vi "Read VI Blocks.vi"(8 "error in (no error)":errorcluster, 11 "Path in (vi, ctl, llb)":path) -> (0 "error out":errorcluster, 1 "Filenames":string[](array[string]), 2 "Blocks":T1(array[cluster]), 3 "Path out":path)   [LabVIEW 2022 SP3]
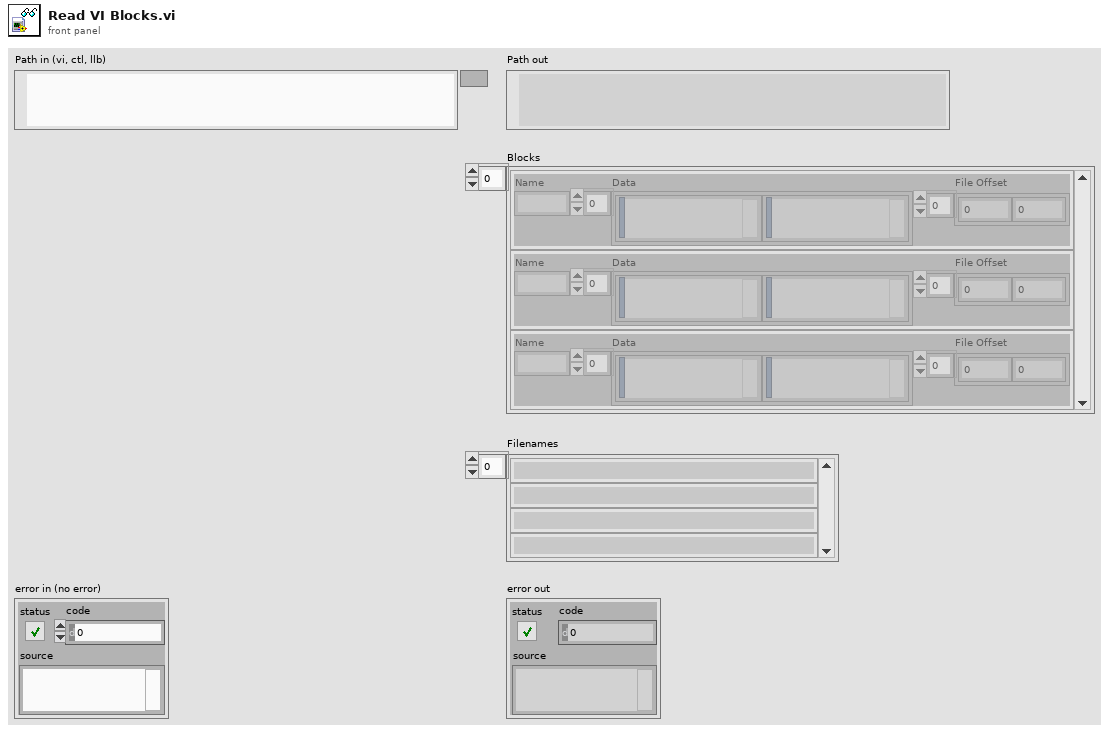
[diagram p1: front panel]
types:
  T1 = cluster{"Name":string, "Data":string[], "File Offset":u32[]}[]
  T2 = cluster{"BLOCK_INFO":cluster{"Int1":i32, "Int2":i32, "Int3":i32, "Offset":u32, "Size":u32}[]}
  T3 = cluster{"Name":string, "Data":string[], "Offset":u32[]}
  T4 = enum16{"open", "replace", "create", "open or create", "replace or create", "replace or create with confirmation"}
  T5 = cluster{"RSRC_Identifier":u64, "RSRC_Type":u32, "RSRC_Creator":u32, "Info_Offset":u32, "Info_Size":u32, "Data_Offset":u32, "Data_Size":u32}
  T6 = cluster{"Int1":i32, "Int2":i32, "Int3":i32, "Offset":u32, "Size":u32}
  T7 = cluster{"Int1":i32, "Int2":i32, "Int3":i32, "Offset":u32, "Size":u32}[]
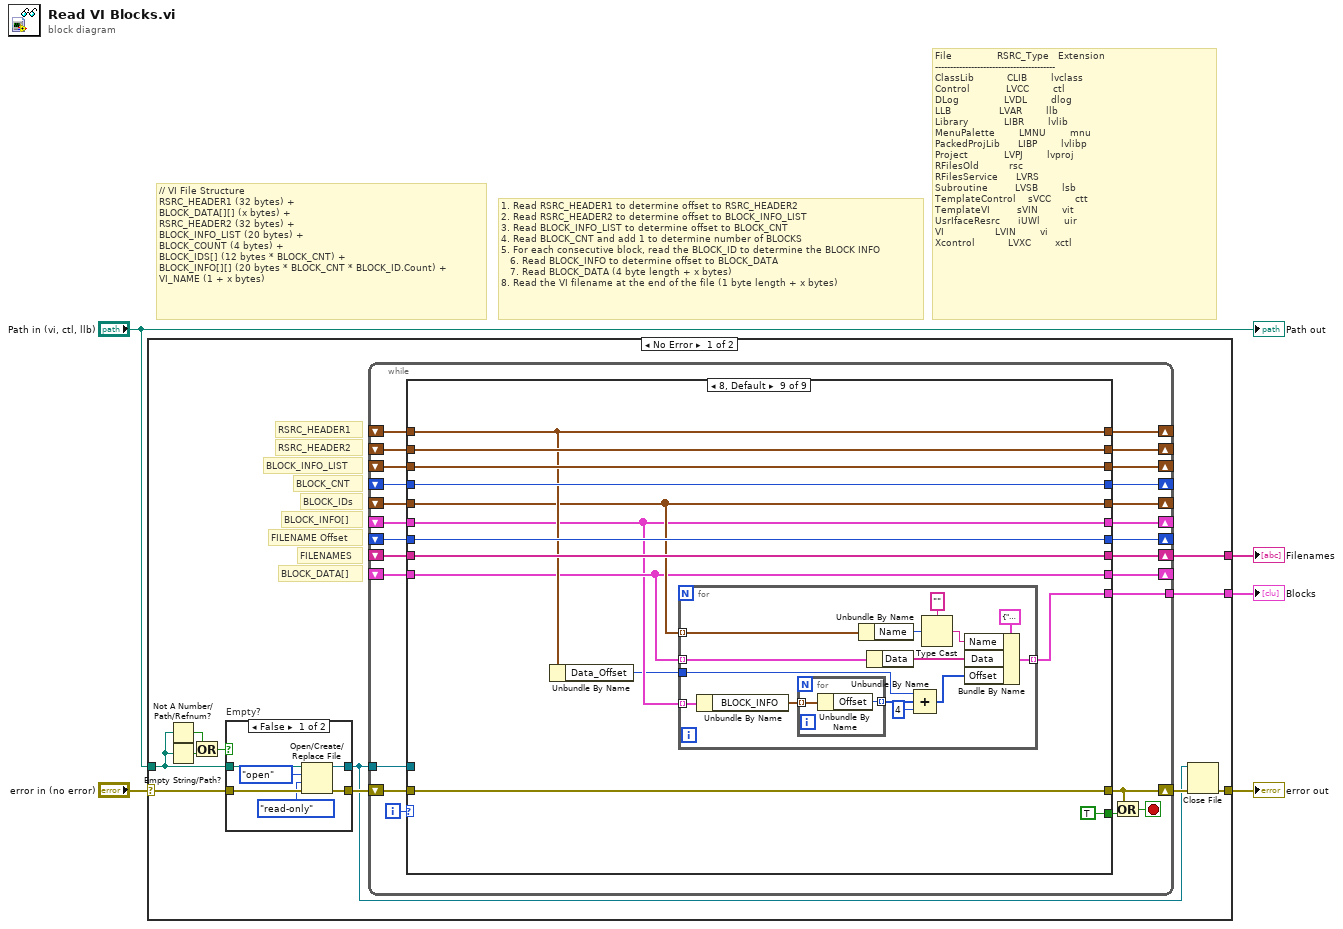
[diagram p0: block diagram]
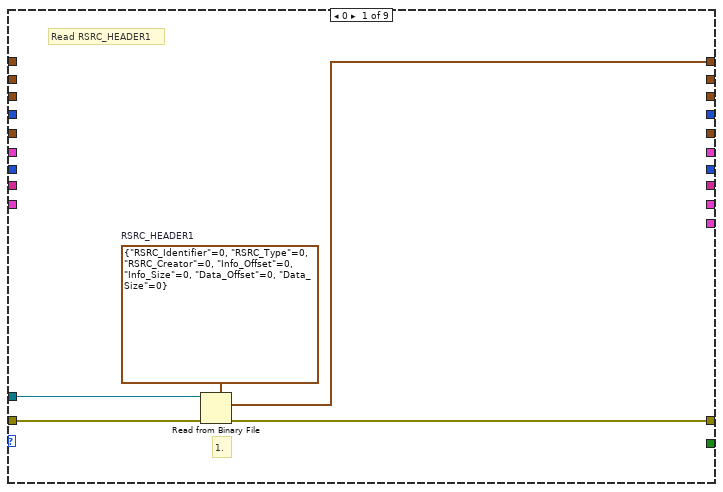
[diagram p2: hidden frame]
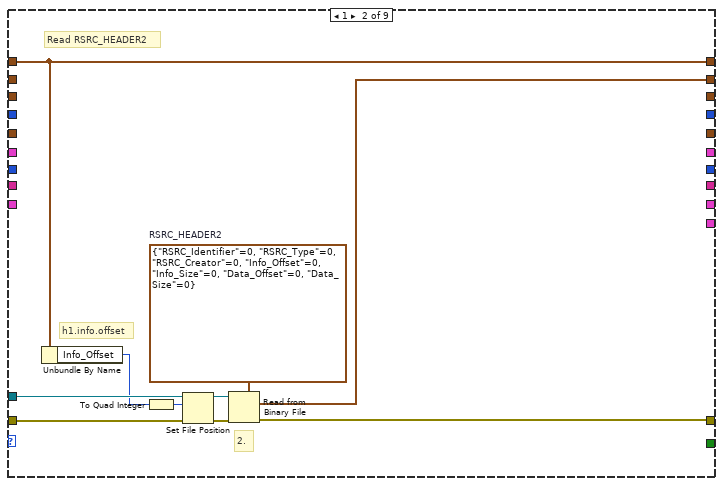
[diagram p3: hidden frame]
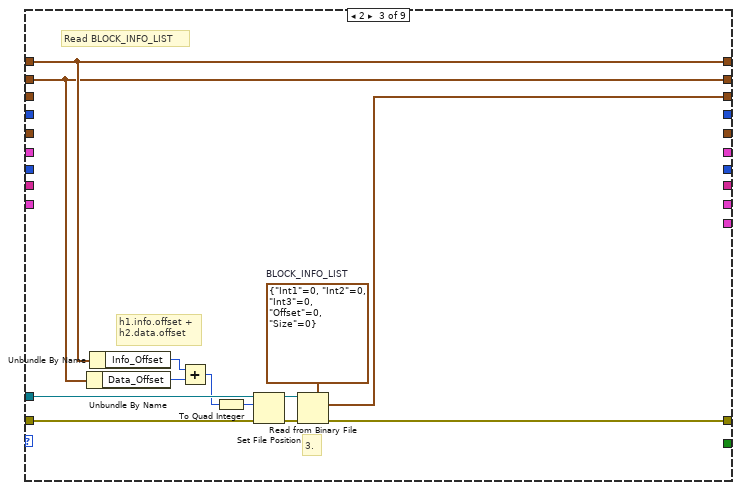
[diagram p4: hidden frame]
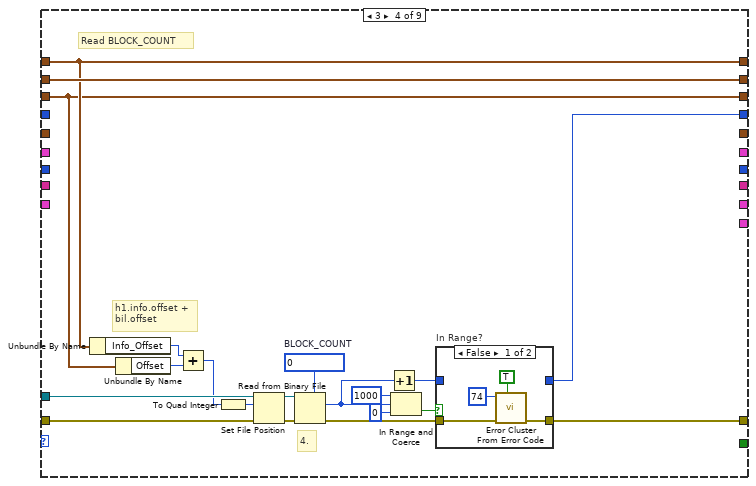
[diagram p5: hidden frame]
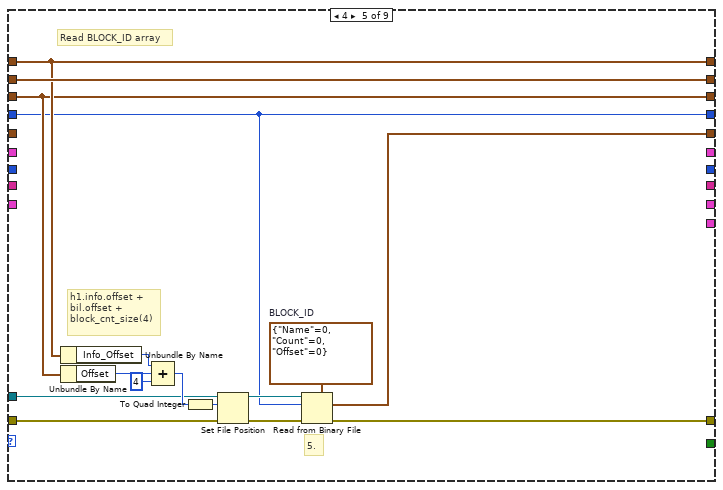
[diagram p7: hidden frame]
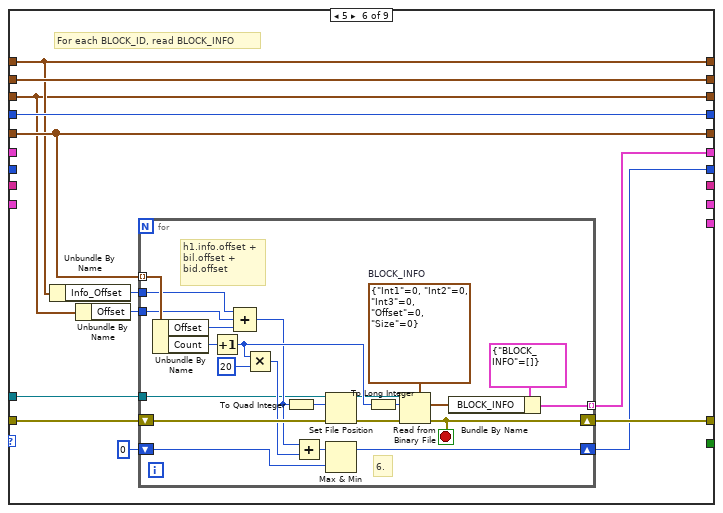
[diagram p8: hidden frame]
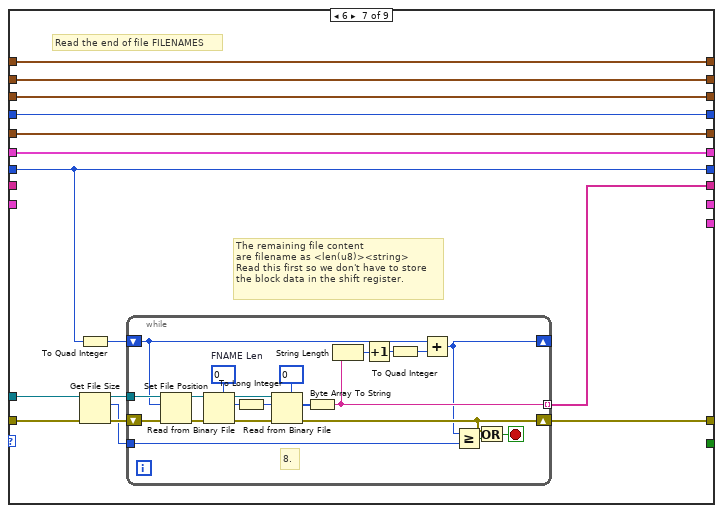
[diagram p9: hidden frame]
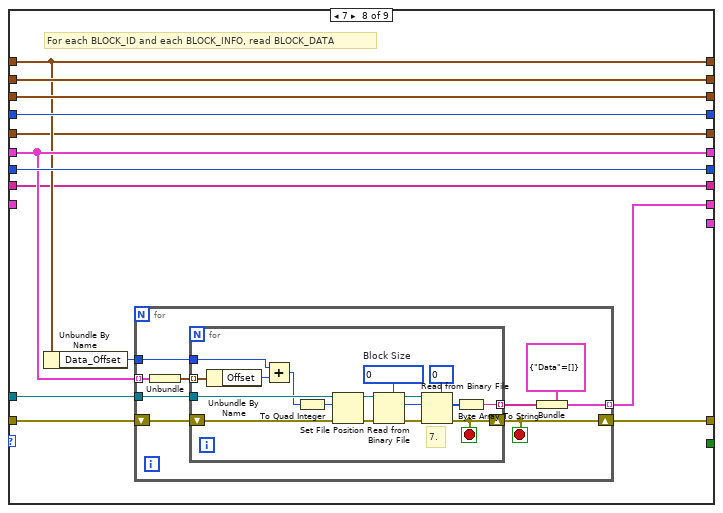
[diagram p10: hidden frame]
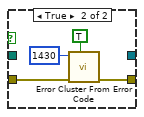
[diagram p11: hidden frame]
diagram:
  # "1. Read RSRC_HEADER1 to determine offset to RSRC_HEADER2\n2. Read RSRC_HEADER2 to determine offset to BLOCK_INFO_LIST\n3. Read BLOCK_INFO_LIST to determine offset to BLOCK_CNT\n4. Read BLOCK_CNT and add 1 to determine number of BLOCKS\n5. For each consecutive block, read the BLOCK_ID to determine the BLOCK INFO\n   6. Read BLOCK_INFO to determine offset to BLOCK_DATA\n   7. Read BLOCK_DATA (4 byte length + x bytes)\n8. Read the VI filename at the end of the file (1 byte length + x bytes)"
  # "// VI File Structure\nRSRC_HEADER1 (32 bytes) + \nBLOCK_DATA[][] (x bytes) +\nRSRC_HEADER2 (32 bytes) + \nBLOCK_INFO_LIST (20 bytes) +\nBLOCK_COUNT (4 bytes) + \nBLOCK_IDS[] (12 bytes * BLOCK_CNT) +\nBLOCK_INFO[][] (20 bytes * BLOCK_CNT * BLOCK_ID.Count) +\nVI_NAME (1 + x bytes)"
  # "File               RSRC_Type   Extension\n----------------------------------------\nClassLib           CLIB        lvclass\nControl            LVCC        ctl\nDLog               LVDL        dlog\nLLB                LVAR        llb\nLibrary            LIBR        lvlib\nMenuPalette        LMNU        mnu\nPackedProjLib      LIBP        lvlibp\nProject            LVPJ        lvproj\nRFilesOld          rsc         \nRFilesService      LVRS        \nSubroutine         LVSB        lsb\nTemplateControl    sVCC        ctt\nTemplateVI         sVIN        vit\nUsrIfaceResrc      iUWl        uir\nVI                 LVIN        vi\nXcontrol           LVXC        xctl"
  n1 = case shown="No Error" "error in (no error)" {
    selector: "error in (no error)" -> [w16 w262]
    tunnel: "Path in (vi, ctl, llb)" -> [w15 _]
    tunnel: [w11 _] -> w4
    tunnel: [w8 w262] -> w3
    tunnel: [w6 _] -> w2
    frame No Error {
      # "BLOCK_DATA[]"
      # "FILENAME Offset"
      # "BLOCK_INFO[]"
      # "BLOCK_IDs"
      # "BLOCK_CNT"
      # "BLOCK_INFO_LIST"
      # "RSRC_HEADER2"
      # "FILENAMES"
      # "RSRC_HEADER1"
      n2 = Not A Number/Path/Refnum?(number/path/refnum=w15) -> (NaN/Path/Refnum?=w13:bool)
      n3 = Empty String/Path?(string/path=w15) -> (empty?=w14:bool)
      n4 = Or(x=w13, y=w14) -> (x .or. y?=w12:bool)
      n5 = case "Empty?" shown="False" w12 {
        tunnel: w16 -> [w257 w261]
        tunnel: w15 -> [w254 _]
        tunnel: [w253 w258] -> w10
        tunnel: [w252 _] -> w7
        frame False {
          n6 = Open/Create/Replace File(file path (use dialog)=w254, error in=w257, operation (0:open)=T4."open", access (0:read/write)=enum16{"read/write", "read-only", "write-only"}."read-only") -> (refnum out=w252:refnum<file>, error out=w253:errorcluster)  [unwired: 2 in, 1 out]
        }
        frame True {
          n7 = call <vilib>:"Error Cluster From Error Code.vi"("show call chain? (False)"=TRUE, "error in (no error)"=w261, "error code (0)"=1430) -> ("error out"=w258:errorcluster)  [unwired: 6 in]
        }
      }
      n8 = while {
        tunnel: w7 -> [w40]
        shift-right: [w36] -> w9
        shift-left: w10 -> [w41]
        shift-right: [w38] -> _
        shift-left: _ -> [w37]
        shift-right: [w33] -> _
        shift-left: _ -> [w32]
        shift-right: [w31] -> _
        shift-left: _ -> [w30]
        shift-right: [w29] -> _
        shift-left: _ -> [w28]
        shift-right: [w27] -> _
        shift-left: _ -> [w26]
        shift-right: [w25] -> _
        shift-left: _ -> [w24]
        shift-right: [w23] -> _
        shift-left: _ -> [w22]
        shift-right: [w20] -> w11
        shift-left: _ -> [w19]
        shift-right: [w21] -> _
        shift-left: _ -> [w18]
        tunnel: [w17] -> w6
        i -> [w39]
        stop <- w35 stop-if-true
        n9 = case shown="8, Default" w39 {
          tunnel: w41 -> [w46 w56 w69 w85 w108 w122 w156 w192 w229]
          tunnel: [w44 w54 w68 w84 w107 w120 w155 w186 w229] -> w36
          tunnel: w40 -> [w45 w51 w61 w74 w99 w121 w152 w188 _]
          tunnel: [w42 w55 w67 w83 w106 w118 w162 w190 w228] -> w38
          tunnel: w37 -> [_ w55 w67 w83 w106 w118 w162 w190 w228]
          tunnel: [_ _ _ _ _ _ _ _ TRUE] -> w34
          tunnel: [_ w53 w66 w89 w111 w124 w161 w196 w235] -> w33
          tunnel: w32 -> [_ _ w66 w89 w111 w124 w161 w196 w235]
          tunnel: [_ _ w63 w82 w105 w117 w160 w195 w234] -> w31
          tunnel: w30 -> [_ _ _ w82 w105 w117 w160 w195 w234]
          tunnel: [_ _ _ w76 w97 w123 w159 w194 w233] -> w29
          tunnel: w28 -> [_ _ _ _ w97 w123 w159 w194 w233]
          tunnel: [_ _ _ _ w96 w119 w158 w187 w227] -> w27
          tunnel: w26 -> [_ _ _ _ _ w119 w158 w187 w227]
          tunnel: [_ _ _ _ _ w113 w157 w191 w224] -> w25
          tunnel: w24 -> [_ _ _ _ _ _ w157 w191 w224]
          tunnel: [_ _ _ _ _ w112 w150 w193 w232] -> w23
          tunnel: w22 -> [_ _ _ _ _ _ w150 w193 w232]
          tunnel: [_ _ _ _ _ _ _ w185 w226] -> w21
          tunnel: [_ _ _ _ _ _ w154 w184 w231] -> w20
          tunnel: w19 -> [_ _ _ _ _ _ _ w184 w231]
          tunnel: w18 -> [_ _ _ _ _ _ _ _ w226]
          tunnel: [_ _ _ _ _ _ _ _ w225] -> w17
          frame 0 {
            w43 = T5 {"RSRC_Identifier"=0, "RSRC_Type"=0, "RSRC_Creator"=0, "Info_Offset"=0, "Info_Size"=0, "Data_Offset"=0, "Data_Size"=0}  # RSRC_HEADER1
            # "Read RSRC_HEADER1"
            # "1."
            n10 = Read from Binary File(5:w43, 8:w46, 11:w45) -> (0:w44:errorcluster, 2:w42:T5)  [unwired: 3 in, 2 out]
          }
          frame 1 {
            w49 = T5 {"RSRC_Identifier"=0, "RSRC_Type"=0, "RSRC_Creator"=0, "Info_Offset"=0, "Info_Size"=0, "Data_Offset"=0, "Data_Size"=0}  # RSRC_HEADER2
            # "Read RSRC_HEADER2"
            # "2."
            # "h1.info.offset"
            n11 = Unbundle By Name(w55) -> ("Info_Offset"=w50:u32)
            n12 = To Quad Integer(1:w50) -> (0:w47:i64)
            n13 = Set File Position(offset (in bytes) (0)=w47, refnum=w51, error in=w56) -> (refnum out=w48:refnum<file>, error out=w52:errorcluster)  [unwired: 1 in]
            n14 = Read from Binary File(5:w49, 8:w52, 11:w48) -> (0:w54:errorcluster, 2:w53:T5)  [unwired: 3 in, 2 out]
          }
          frame 2 {
            w60 = T6 {"Int1"=0, "Int2"=0, "Int3"=0, "Offset"=0, "Size"=0}  # BLOCK_INFO_LIST
            # "Read BLOCK_INFO_LIST"
            # "3."
            # "h1.info.offset +\nh2.data.offset"
            n15 = Unbundle By Name(w66) -> ("Data_Offset"=w65:u32)
            n16 = Unbundle By Name(w67) -> ("Info_Offset"=w64:u32)
            n17 = Add(x=w64, y=w65) -> (x+y=w58:u32)
            n18 = To Quad Integer(1:w58) -> (0:w57:i64)
            n19 = Set File Position(offset (in bytes) (0)=w57, refnum=w61, error in=w69) -> (refnum out=w59:refnum<file>, error out=w62:errorcluster)  [unwired: 1 in]
            n20 = Read from Binary File(5:w60, 8:w62, 11:w59) -> (0:w68:errorcluster, 2:w63:T6)  [unwired: 3 in, 2 out]
          }
          frame 3 {
            w73 = 0  # BLOCK_COUNT
            # "Read BLOCK_COUNT"
            # "4."
            # "h1.info.offset +\nbil.offset"
            n21 = Unbundle By Name(w83) -> ("Info_Offset"=w80:u32)
            n22 = Unbundle By Name(w82) -> ("Offset"=w81:u32)
            n23 = Add(x=w80, y=w81) -> (x+y=w71:u32)
            n24 = To Quad Integer(1:w71) -> (0:w70:i64)
            n25 = Set File Position(offset (in bytes) (0)=w70, refnum=w74, error in=w85) -> (refnum out=w72:refnum<file>, error out=w75:errorcluster)  [unwired: 1 in]
            n26 = Read from Binary File(5:w73, 8:w75, 11:w72) -> (0:w86:errorcluster, 2:w77:i32)  [unwired: 3 in, 2 out]
            n27 = Increment(x=w77) -> (x+1=w78:i32)
            n28 = In Range and Coerce(upper limit=1000, x=w77, lower limit=0) -> (In Range?=w79:bool)  [unwired: 1 out]
            n29 = case "In Range?" shown="False" w79 {
              tunnel: w86 -> [w91 w95]
              tunnel: [w90 w95] -> w84
              tunnel: w78 -> [_ w94]
              tunnel: [_ w94] -> w76
              frame False {
                n30 = call <vilib>:"Error Cluster From Error Code.vi"("show call chain? (False)"=TRUE, "error in (no error)"=w91, "error code (0)"=74) -> ("error out"=w90:errorcluster)  [unwired: 6 in]
              }
              frame True {
              }
            }
          }
          frame 4 {
            w101 = cluster{"Name":u32, "Count":u32, "Offset":u32} {"Name"=0, "Count"=0, "Offset"=0}  # BLOCK_ID
            # "Read BLOCK_ID array"
            # "5."
            # "h1.info.offset +\nbil.offset +\nblock_cnt_size(4)"
            n31 = Unbundle By Name(w106) -> ("Info_Offset"=w110:u32)
            n32 = Unbundle By Name(w105) -> ("Offset"=w109:u32)
            n33 = Compound Arithmetic op=ADD(w110, w109, u32 4 ("value")) -> (w100:u32)
            n34 = To Quad Integer(1:w100) -> (0:w98:i64)
            n35 = Set File Position(offset (in bytes) (0)=w98, refnum=w99, error in=w108) -> (refnum out=w102:refnum<file>, error out=w103:errorcluster)  [unwired: 1 in]
            n36 = Read from Binary File(5:w101, 8:w103, 10:w97, 11:w102) -> (0:w107:errorcluster, 2:w96:cluster{"Name":u32, "Count":u32, "Offset":u32}[])  [unwired: 2 in, 2 out]
          }
          frame 5 {
            # "For each BLOCK_ID, read BLOCK_INFO"
            n37 = Unbundle By Name(w118) -> ("Info_Offset"=w116:u32)
            n38 = Unbundle By Name(w117) -> ("Offset"=w115:u32)
            n39 = for {
              tunnel: w121 -> [w127]
              shift-right: [w134] -> w120
              shift-left: w122 -> [w147]
              tunnel: w119 -> [w146] mode=indexing
              tunnel: w116 -> [w142]
              tunnel: w115 -> [w141]
              shift-right: [w138] -> w112
              shift-left: u32 0 -> [w137]
              tunnel: [w135] -> w113 mode=indexing
              stop <- w134 stop-if-true
              w133 = T6 {"Int1"=0, "Int2"=0, "Int3"=0, "Offset"=0, "Size"=0}  # BLOCK_INFO
              # "6."
              # "h1.info.offset +\nbil.offset +\nbid.offset"
              n40 = Unbundle By Name(w146) -> ("Offset"=w143:u32, "Count"=w144:u32)
              n41 = Increment(x=w144) -> (x+1=w132:u32)
              n42 = Compound Arithmetic op=ADD(w142, w141, w143) -> (w128:u32)
              n43 = Multiply(x=w132, y=u32 20 ("length (rest)")) -> (x*y=w140:u32)
              n44 = To Quad Integer(1:w128) -> (0:w126:i64)
              n45 = Add(x=w128, y=w140) -> (x+y=w139:u32)
              n46 = Set File Position(offset (in bytes) (0)=w126, refnum=w127, error in=w147) -> (refnum out=w130:refnum<file>, error out=w131:errorcluster)  [unwired: 1 in]
              n47 = Max & Min(x=w139, y=w137) -> (max(x,y)=w138:u32)  [unwired: 1 out]
              n48 = To Long Integer(number=w132) -> (32bit integer=w129:i32)
              n49 = Read from Binary File(5:w133, 8:w131, 10:w129, 11:w130) -> (0:w134:errorcluster, 2:w136:T7)  [unwired: 2 in, 2 out]
              n50 = Bundle By Name(cluster=T2 {"BLOCK_INFO"=[]}, "BLOCK_INFO"=w136) -> (w135:T2)
            }
          }
          frame 6 {
            # "Read the end of file FILENAMES"
            # "The remaining file content\nare filename as <len(u8)><string>\nRead this first so we don't have to store\nthe block data in the shift register."
            n51 = To Quad Integer(1:w150) -> (0:w149:i64)
            n52 = Get File Size(file=w152, error in=w156) -> (refnum out=w151:refnum<file>, size (in bytes)=w148:i64, 0:w153:errorcluster)
            n53 = while {
              tunnel: [w172] -> w154 mode=indexing
              tunnel: w151 -> [w181]
              shift-right: [w170] -> w155
              shift-left: w153 -> [w183]
              shift-right: [w165] -> _
              shift-left: w149 -> [w166]
              tunnel: w148 -> [w164]
              stop <- w169 stop-if-true
              w178 = u8 0  # FNAME Len
              # "8."
              n54 = Set File Position(offset (in bytes) (0)=w166, refnum=w181, error in=w183) -> (refnum out=w180:refnum<file>, error out=w182:errorcluster)  [unwired: 1 in]
              n55 = Read from Binary File(5:w178, 8:w182, 11:w180) -> (0:w179:errorcluster, 2:w175:u8, 3:w176:refnum<file>)  [unwired: 3 in, 1 out]
              n56 = To Long Integer(number=w175) -> (32bit integer=w174:i32)
              n57 = Read from Binary File(5:u8 0, 8:w179, 10:w174, 11:w176) -> (0:w170:errorcluster, 2:w173:u8[])  [unwired: 2 in, 2 out]
              n58 = Byte Array To String(unsigned byte array=w173) -> (string=w172:string)
              n59 = String Length(string=w172) -> (length=w171:i32)
              n60 = Increment(x=w171) -> (x+1=w168:i32)
              n61 = To Quad Integer(1:w168) -> (0:w167:i64)
              n62 = Add(x=w166, y=w167) -> (x+y=w165:i64)
              n63 = Greater Or Equal?(x=w165, y=w164) -> (x >= y?=w163:bool)
              n64 = Or(x=w170, y=w163) -> (x .or. y?=w169:bool)
            }
          }
          frame 7 {
            # "For each BLOCK_ID and each BLOCK_INFO, read BLOCK_DATA"
            n65 = Unbundle By Name(w190) -> ("Data_Offset"=w189:u32)
            n66 = for {
              tunnel: w191 -> [w204] mode=indexing
              tunnel: w189 -> [w202]
              tunnel: w188 -> [w201]
              shift-right: [w200] -> w186
              shift-left: w192 -> [w205]
              tunnel: [w198] -> w185 mode=indexing
              stop <- w200 stop-if-true
              n67 = Unbundle(w204) -> ("BLOCK_INFO"=w203:T7)
              n68 = for {
                tunnel: w201 -> [w215]
                shift-right: [w217] -> w200
                shift-left: w205 -> [w222]
                tunnel: [w206] -> w199 mode=indexing
                tunnel: w203 -> [w219] mode=indexing
                tunnel: w202 -> [w218]
                stop <- w217 stop-if-true
                w209 = 0  # Block Size
                # "7."
                n69 = Unbundle By Name(w219) -> ("Offset"=w221:u32)
                n70 = Add(x=w218, y=w221) -> (x+y=w214:u32)
                n71 = To Quad Integer(1:w214) -> (0:w213:i64)
                n72 = Set File Position(offset (in bytes) (0)=w213, refnum=w215, error in=w222) -> (refnum out=w211:refnum<file>, error out=w216:errorcluster)  [unwired: 1 in]
                n73 = Read from Binary File(5:w209, 8:w216, 11:w211) -> (0:w212:errorcluster, 2:w207:i32, 3:w210:refnum<file>)  [unwired: 3 in, 1 out]
                n74 = Read from Binary File(5:u8 0, 8:w212, 10:w207, 11:w210) -> (0:w217:errorcluster, 2:w220:u8[])  [unwired: 2 in, 2 out]
                n75 = Byte Array To String(unsigned byte array=w220) -> (string=w206:string)
              }
              n76 = Bundle(cluster=cluster{"Data":string[]} {"Data"=[]}, "Data"=w199) -> (w198:cluster{"Data":string[]})
            }
          }
          frame 8, Default {
            n77 = Unbundle By Name(w228) -> ("Data_Offset"=w223:u32)
            n78 = for {
              tunnel: w227 -> [w248] mode=indexing
              tunnel: [w244] -> w225 mode=indexing
              tunnel: w226 -> [w243] mode=indexing
              tunnel: w224 -> [w241] mode=indexing
              tunnel: w223 -> [w236]
              n79 = Unbundle By Name(w241) -> ("BLOCK_INFO"=w240:T7)
              n80 = for {
                tunnel: w240 -> [w251] mode=indexing
                tunnel: [w250] -> w239 mode=indexing
                n81 = Unbundle By Name(w251) -> ("Offset"=w250:u32)
              }
              n82 = Unbundle By Name(w248) -> ("Name"=w247:u32)
              n83 = Unbundle By Name(w243) -> ("Data"=w242:string[])
              n84 = Compound Arithmetic op=ADD(w236, w239, u32 4 ("value")) -> (w237:u32[])
              n85 = Type Cast(type="", x=w247) -> (*(type *) &x=w246:string)
              n86 = Bundle By Name(cluster=T3 {"Name"="", "Data"=[], "Offset"=[]} ("Block"), "Name"=w246, "Data"=w242, "Offset"=w237) -> (w244:T3)
            }
          }
        }
        n87 = Or(x=w36, y=w34) -> (x .or. y?=w35:bool)
      }
      n88 = Close File(refnum=w7, error in=w9) -> (error out=w8:errorcluster)  [unwired: 1 out]
    }
    frame Error {
    }
  }
  "error out" <- w3
  "Filenames" <- w4
  "Blocks" <- w2
  "Path out" <- "Path in (vi, ctl, llb)"
